vi "test_CCDSetAndGetAcquisitionCount.vi"(7 "Test should pass":bool=TRUE, 8 "error in":errorcluster, 9 "tear down connection":bool=TRUE, 10 "set-up a connection":bool=TRUE, 11 "device selection":enum16{"monochromator", "CCD", "SCD"}(ring)=enum."CCD") -> (0 "error out":errorcluster)   [LabVIEW 2023]
uses:
  Source/Classes/Mono/Monochromator.lvclass
  Source/Classes/CCD/CCD.lvclass
  Source/Classes/SCD/SCD.lvclass
  <vilib>/addons/_JKI Toolkits/Caraya/classes/Assert/Assert Equal Value and Type_Variant.vi
  <vilib>/addons/_JKI Toolkits/Caraya/classes/Assert/Assert Not Error.vi
  Source/Classes/GenericDevice/GenericDevice.lvclass
  <vilib>/addons/_JKI Toolkits/Caraya/classes/Test/Test.lvclass
  <vilib>/addons/_JKI Toolkits/Caraya/classes/Assert/Assert.lvclass
  C:/Users/grju/Desktop/AbgelegteDokumente/Kunden/Horiba/horiba-labview-sdk/Source/Classes/GenericDevice/GenericDevice.lvclass
  C:/Users/grju/Desktop/AbgelegteDokumente/Kunden/Horiba/horiba-labview-sdk/Source/Classes/CCD/CCD.lvclass
panel:
  # "Connector Pane"
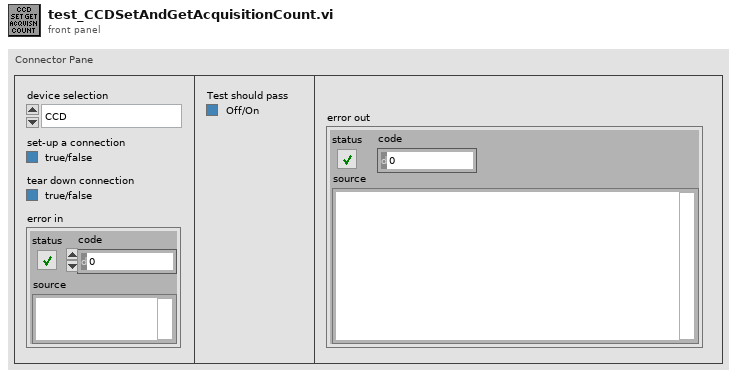
[diagram p1: front panel]
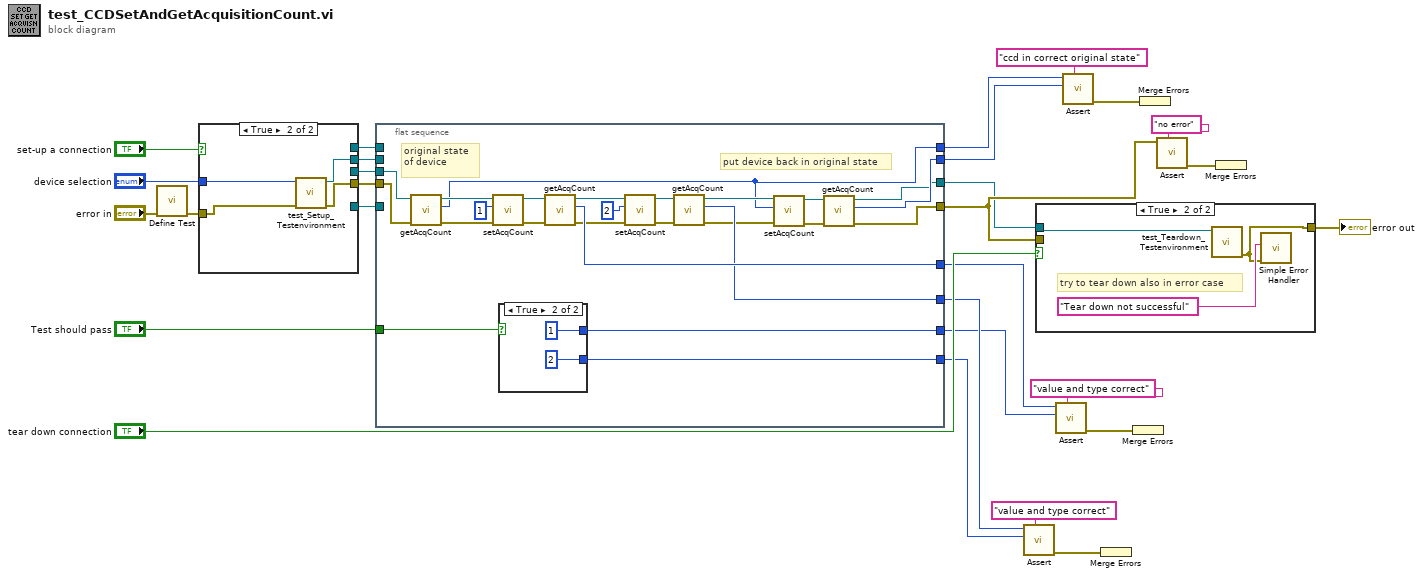
[diagram p0: block diagram]
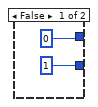
[diagram p2: hidden frame]
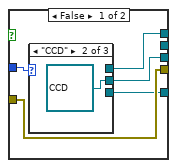
[diagram p3: hidden frame]
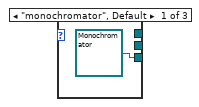
[diagram p4: hidden frame]
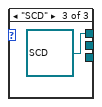
[diagram p5: hidden frame]
diagram:
  n1 = call <vilib>:"Define Test.vi"("error in (no error)"="error in") -> ("error out"=w20:errorcluster)  [unwired: 9 in, 1 out]
  n2 = case shown="True" "set-up a connection" {
    tunnel: w20 -> [w33 w40]
    tunnel: [w33 w39] -> w22
    tunnel: "device selection" -> [w32 w38]
    tunnel: [_ w37] -> w19
    tunnel: [w31 _] -> w18
    tunnel: [w30 _] -> w17
    tunnel: [w29 _] -> w16
    frame False {
      n3 = case shown="\"CCD\"" w32 {
        tunnel: [refnum<class "Monochromator.lvclass"> refnum ("Monochromator.lvclass") _ _] -> w31
        tunnel: [_ refnum<class "CCD.lvclass"> refnum ("CCD in") _] -> w30
        tunnel: [_ _ refnum<class "SCD.lvclass"> refnum ("SCD.lvclass")] -> w29
        frame "monochromator", Default {
        }
        frame "CCD" {
        }
        frame "SCD" {
        }
      }
    }
    frame True {
      n4 = call "test_Setup_Testenvironment.vi"("error in"=w40, "device selection"=w38) -> ("error out"=w39:errorcluster, "GenericDevice.lvclass"=w37:refnum<class "GenericDevice.lvclass">)  [unwired: 7 in, 1 out]
    }
  }
  n5 = flat-sequence {
    tunnel: w22 -> [w61]
    tunnel: w19 -> [_]
    tunnel: w18 -> [_]
    tunnel: w17 -> [w62]
    tunnel: w16 -> [_]
    tunnel: [w41] -> w11
    tunnel: "Test should pass" -> [w65]
    tunnel: [w42] -> w10
    tunnel: [w49] -> w9
    tunnel: [w64] -> w8
    tunnel: [w55] -> w7
    tunnel: [w63] -> w6
    tunnel: [w44] -> w3
    tunnel: [w43] -> w2
    frame #0 {
      # "put device back in original state"
      # "original state of device"
      n6 = call "getAcqCount.vi"("error in (no error)"=w61, "CCD in"=w62) -> ("error out"=w59:errorcluster, "count"=w44:i32, "CCD out"=w60:refnum<class "CCD.lvclass">)  [unwired: 7 in]
      n7 = call "setAcqCount.vi"("error in (no error)"=w59, "count"=1 ("exposure time [ms]"), "CCD in"=w60) -> ("error out"=w57:errorcluster, "CCD out"=w56:refnum<class "CCD.lvclass">)  [unwired: 5 in, 2 out]
      n8 = case shown="True" w65 {
        tunnel: [1 ("exposure time [ms]") 2 ("exposure time [ms]")] -> w64
        tunnel: [0 ("exposure time [ms]") 1 ("exposure time [ms]")] -> w63
        frame False {
        }
        frame True {
        }
      }
      n9 = call "getAcqCount.vi"("error in (no error)"=w57, "CCD in"=w56) -> ("error out"=w51:errorcluster, "count"=w55:i32, "CCD out"=w52:refnum<class "CCD.lvclass">)  [unwired: 7 in]
      n10 = call "setAcqCount.vi"("error in (no error)"=w51, "count"=2 ("exposure time [ms]"), "CCD in"=w52) -> ("error out"=w54:errorcluster, "CCD out"=w53:refnum<class "CCD.lvclass">)  [unwired: 5 in, 2 out]
      n11 = call "getAcqCount.vi"("error in (no error)"=w54, "CCD in"=w53) -> ("error out"=w46:errorcluster, "count"=w49:i32, "CCD out"=w47:refnum<class "CCD.lvclass">)  [unwired: 7 in]
      n12 = call "setAcqCount.vi"("error in (no error)"=w46, "count"=w44, "CCD in"=w47) -> ("error out"=w48:errorcluster, "CCD out"=w45:refnum<class "CCD.lvclass">)  [unwired: 5 in, 2 out]
      n13 = call "getAcqCount.vi"("error in (no error)"=w48, "CCD in"=w45) -> ("error out"=w41:errorcluster, "count"=w43:i32, "CCD out"=w42:refnum<class "CCD.lvclass">)  [unwired: 7 in]
    }
  }
  n14 = call-poly <vilib>:"Assert.vi"("Label"="value and type correct" ("Label (VI Title)"), "Y"=w8, "X"=w9) -> ("error out"=w26:errorcluster)  [unwired: 7 in, 1 out]
  n15 = case shown="True" "tear down connection" {
    tunnel: w10 -> [_ w72]
    tunnel: [w70 w71] -> w1
    tunnel: w11 -> [w70 _]
    frame False {
    }
    frame True {
      # "try to tear down also in error case"
      n16 = call "test_Teardown_Testenvironment.vi"("GenericDevice.lvclass"=w72) -> ("error out"=w71:errorcluster)  [unwired: 9 in, 1 out]
      n17 = call <vilib>:"Simple Error Handler.vi"("error source (\" \")"="Tear down not successful" ("error source (\" \")"), "error in (no error)"=w71) -> ()  [unwired: 3 in, 5 out]
    }
  }
  "error out" <- w1
  n18 = call-poly <vilib>:"Assert.vi"("Label"="value and type correct" ("Label (VI Title)"), "Y"=w6, "X"=w7) -> ("error out"=w24:errorcluster)  [unwired: 7 in, 1 out]
  n19 = call-poly <vilib>:"Assert.vi"("Label"="ccd in correct original state" ("Label (VI Title)"), "Y"=w2, "X"=w3) -> ("error out"=w5:errorcluster)  [unwired: 7 in, 1 out]
  n20 = Merge Errors(w26) -> ()  [unwired: 1 out]
  n21 = Merge Errors(w24) -> ()  [unwired: 1 out]
  n22 = Merge Errors(w5) -> ()  [unwired: 1 out]
  n23 = call-poly <vilib>:"Assert.vi"("Label"="no error" ("Label (VI Title)"), "Not Error?"=w11) -> ("error out"=w13:errorcluster)  [unwired: 8 in, 1 out]
  n24 = Merge Errors(w13) -> ()  [unwired: 1 out]
